vi "Register For Hotel.vi"(9 "hotel":string, 10 "guest":string, 11 "map in":map{string, set{string}}(c390)) -> (1 "first registration for this hotel?":bool, 2 "guest already registered here?":bool, 3 "map out":map{string, set{string}}(c390))   [LabVIEW 2023]
doc: "This VI registers a guest for the given hotel."
uses:
  1e01f290-8c99-4c7e-aa8f-4bec2ca940a0.vi
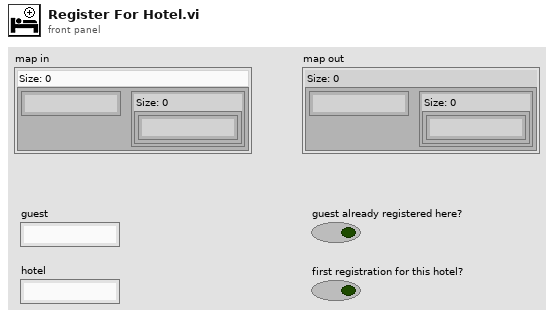
[diagram p1: front panel]
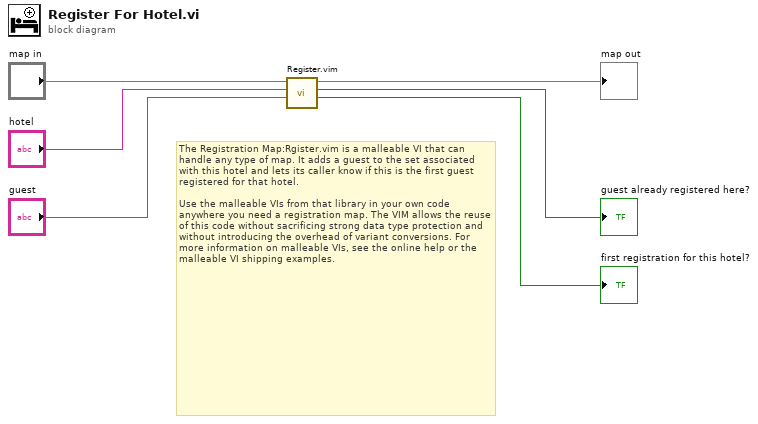
[diagram p0: block diagram]
diagram:
  # "The Registration Map:Rgister.vim is a malleable VI that can handle any type of map. It adds a guest to the set associated with this hotel and lets its caller know if this is the first guest registered for that hotel. \n\nUse the malleable VIs from that library in your own code anywhere you need a registration map. The VIM allows the reuse of this code without sacrificing strong data type protection and without introducing the overhead of variant conversions. For more information on malleable VIs, see the online help or the malleable VI shipping examples."
  n1 = call "Register.vim"("set element"="guest", "key"="hotel", "map in"="map in") -> ("first registration for this key?"=→"first registration for this hotel?":bool, "element already registered?"=→"guest already registered here?":bool, "map out"=→"map out":map{string, set{string}})  [unwired: 6 in]
